vi "Ramping.vi"(1 "Motor Powers":cluster{"RMotor":dbl, "LMotor":dbl}) -> (0 "Motor Powers":cluster{"RMotor":dbl, "LMotor":dbl})   [LabVIEW 2014]
panel:
  in  "Max Change":dbl=0.2
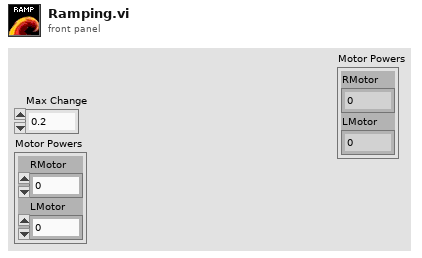
[diagram p1: front panel]
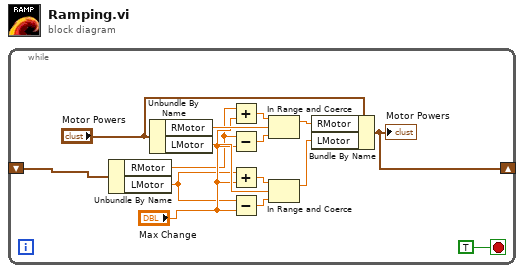
[diagram p0: block diagram]
diagram:
  n1 = while {
    shift-right: [w6] -> _
    shift-left: _ -> [w1]
    stop <- TRUE stop-if-true
    n2 = Unbundle By Name(w1) -> ("RMotor"=w2:dbl, "LMotor"=w3:dbl)
    n3 = Unbundle By Name("Motor Powers") -> ("RMotor"=w11:dbl, "LMotor"=w10:dbl)
    n4 = Add(x=w2, y="Max Change") -> (x+y=w15:dbl)
    n5 = Subtract(x=w2, y="Max Change") -> (x-y=w14:dbl)
    n6 = Add(x=w3, y="Max Change") -> (x+y=w12:dbl)
    n7 = Subtract(x=w3, y="Max Change") -> (x-y=w13:dbl)
    n8 = In Range and Coerce(upper limit=w15, x=w11, lower limit=w14) -> (coerced(x)=w9:dbl)  [unwired: 1 out]
    n9 = In Range and Coerce(upper limit=w12, x=w10, lower limit=w13) -> (coerced(x)=w8:dbl)  [unwired: 1 out]
    n10 = Bundle By Name(cluster="Motor Powers", "RMotor"=w9, "LMotor"=w8) -> (w6:cluster{"RMotor":dbl, "LMotor":dbl})
    "Motor Powers" <- w6
  }
